vi "Get_Reference_API.vi"(0 "DVR":refnum<data-value>, 5 "Subpanel Ref":refnum<vi>, 11 "Error In":errorcluster) -> (4 "DVR Out":refnum<data-value>, 15 "Error Out":errorcluster)   [LabVIEW 2020, in "Test.lvclass"]
doc: "API to get values from the previous loaded subVI"
uses:
  Test.lvclass
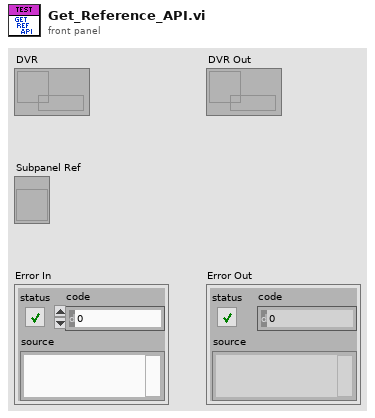
[diagram p1: front panel]
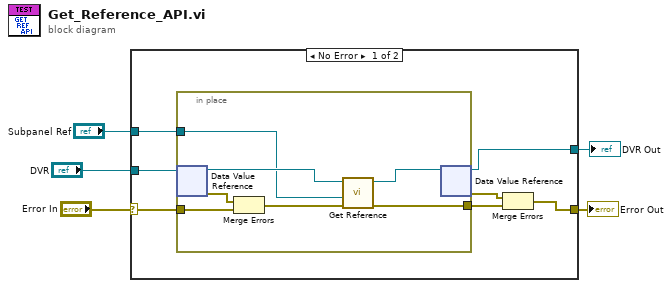
[diagram p0: block diagram]
diagram:
  n1 = case shown="No Error" "Error In" {
    selector: "Error In" -> [w12 w20]
    tunnel: "DVR" -> [w11 w21]
    tunnel: "Subpanel Ref" -> [w10 _]
    tunnel: [w6 w21] -> w2
    tunnel: [w7 w20] -> w1
    frame No Error {
      n2 = in-place {
        in-place-border: w12 -> [w17]
        in-place-border: w10 -> [w15]
        in-place-border: [w13] -> w9
        n3 = in-place-dvr #1(w11) -> (w19:refnum<class "Test.lvclass">, w18:errorcluster)
        n4 = Merge Errors(w18, w17) -> (w16:errorcluster)
        n5 = call-dynamic "Get Reference.vi"("Error In"=w16, "Subpanel Ref"=w15, "Test in"=w19) -> ("Error Out"=w13:errorcluster, "Test out"=w14:refnum<class "Test.lvclass">)  [unwired: 7 in]
        n6 = in-place-dvr #1(w14) -> (w6:refnum<data-value>, w8:errorcluster)
      }
      n7 = Merge Errors(w8, w9) -> (w7:errorcluster)
    }
    frame Error {
    }
  }
  "DVR Out" <- w2
  "Error Out" <- w1
